vi "isHomed.vi"(5 "Device in":refnum<k24>) -> (2 "Device out":refnum<k24>)   [LabVIEW 2014]
doc: "André Romero - 2017\nandretec@ifsc.usp.br"
uses:
  C:/UserLab/andre/GITs/andretec/Thorlabs-Vector-Move/kinesisTec/Kinesis/Thorlabs.MotionControl.TCube.DCServoCLI.dll
  Kinesis/Thorlabs.MotionControl.TCube.DCServoCLI.dll
  C:/UserLab/andre/GITs/andretec/Thorlabs-Vector-Move/kinesisTec/Kinesis/Thorlabs.MotionControl.GenericMotorCLI.dll
  Kinesis/Thorlabs.MotionControl.GenericMotorCLI.dll
  motorsGlobalVar.vi
panel:
  out "IsHomed":bool
  out "SerialNumber":u32
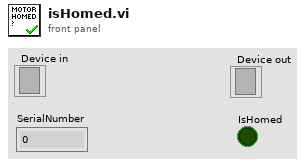
[diagram p1: front panel]
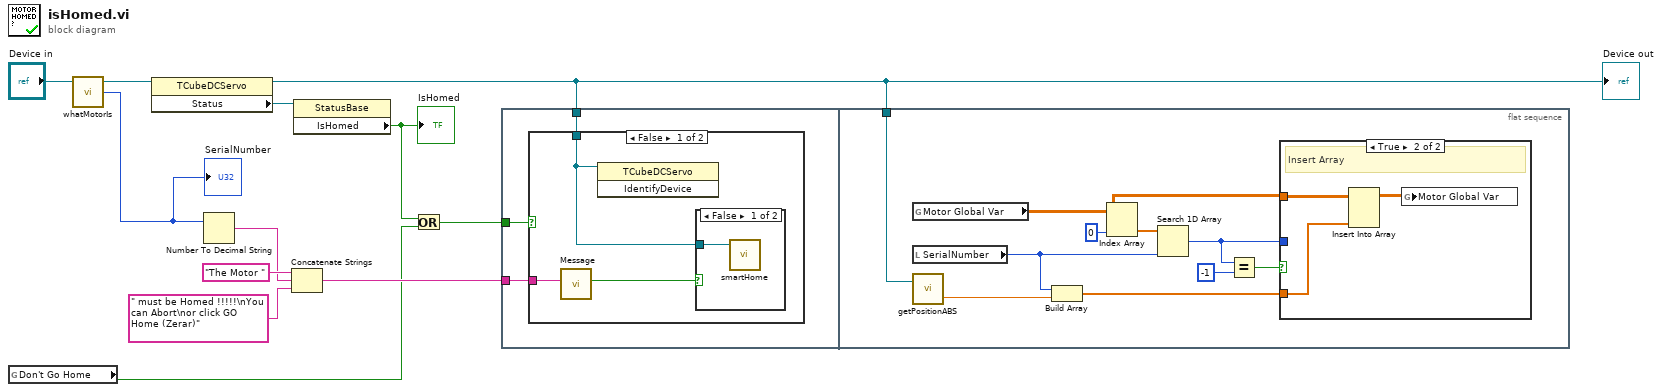
[diagram p0: block diagram]
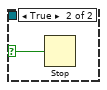
[diagram p2: hidden frame]
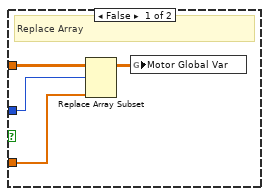
[diagram p4: hidden frame]
diagram:
  n1 = global read "motorsGlobalVar.vi" "Don't Go Home"() -> (w1:bool)
  n2 = call "whatMotorIs.vi"("Device in"="Device in") -> ("SerialNumber"=w10:u32, "Device out"=w4:refnum<k24>)  [unwired: 3 in]
  "SerialNumber" <- w10
  n3 = property class="TCubeDCServo"(reference=w4) -> (reference out=w3:refnum<k24>, "Status"=w11:refnum<k24>)  [unwired: 1 in, 1 out]
  "Device out" <- w3
  n4 = Number To Decimal String(number=w10) -> (decimal integer string=w8:string)  [unwired: 1 in]
  n5 = Concatenate Strings("The Motor ", w8, " must be Homed !!!!!\nYou can Abort\nor click GO Home (Zerar)" ("string")) -> (w6:string)
  n6 = property class="StatusBase"(reference=w11) -> ("IsHomed"=w12:bool)  [unwired: 1 in, 2 out]
  "IsHomed" <- w12
  n7 = Or(x=w12, y=w1) -> (x .or. y?=w2:bool)
  n8 = flat-sequence {
    tunnel: w2 -> [w15]
    tunnel: w6 -> [w14]
    tunnel: w3 -> [w13]
    tunnel: w3 -> [w24]
    frame #0 {
      n9 = case shown="False" w15 {
        tunnel: w14 -> [w18 _]
        tunnel: w13 -> [w16 _]
        frame False {
          n10 = call "Message"("Message"=w18) -> ("Abort"=w17:bool)  [unwired: 9 in, 1 out]
          n11 = invoke class="TCubeDCServo" method="IdentifyDevice"(reference=w16) -> ()  [unwired: 2 in, 3 out]
          n12 = case shown="False" w17 {
            selector: w17 -> [_ w20]
            tunnel: w16 -> [w19 _]
            frame False {
              n13 = call "smartHome.vi"("Device in"=w19) -> ()  [unwired: 4 in, 1 out]
            }
            frame True {
              n14 = Stop(stop? (T)=w20) -> ()
            }
          }
        }
        frame True {
        }
      }
    }
    frame #1 {
      n15 = global read "motorsGlobalVar.vi" "Motor Global Var"() -> (w25:dbl[][])
      n16 = local read "SerialNumber"() -> (w23:u32)
      n17 = call "getPositionABS.vi"("Device"=w24) -> ("GetPOS"=w21:dbl)  [unwired: 1 in, 1 out]
      n18 = Build Array(w23, w21) -> (w22:dbl[])
      n19 = Index Array(array=w25, index (col)=0 ("disabled index (col)")) -> (element=w29:dbl[])  [unwired: 1 in]
      n20 = Search 1D Array(1D array=w29, element=w23) -> (index of element=w26:i32)  [unwired: 1 in]
      n21 = Equal?(x=w26, y=-1) -> (x = y?=w27:bool)
      n22 = case shown="True" w27 {
        tunnel: w26 -> [w33 _]
        tunnel: w25 -> [w34 w37]
        tunnel: w22 -> [w32 w36]
        frame False {
          # "Replace Array"
          n23 = Replace Array Subset(array=w34, new element=w32, index (row)=w33) -> (w31:dbl[][])  [unwired: 1 in]
          n24 = global write "motorsGlobalVar.vi" "Motor Global Var"(w31) -> ()
        }
        frame True {
          # "Insert Array"
          n25 = Insert Into Array(array=w37, new element=w36) -> (w35:dbl[][])  [unwired: 2 in]
          n26 = global write "motorsGlobalVar.vi" "Motor Global Var"(w35) -> ()
        }
      }
    }
  }
